vi "Alarma_Auto.vi"() -> ()   [LabVIEW 2020]
panel:
  in  "Boton3":bool
  out "Alarma":bool
  in  "Boton2":bool
  in  "Boton1":bool
  # "Compuertas Logicas"
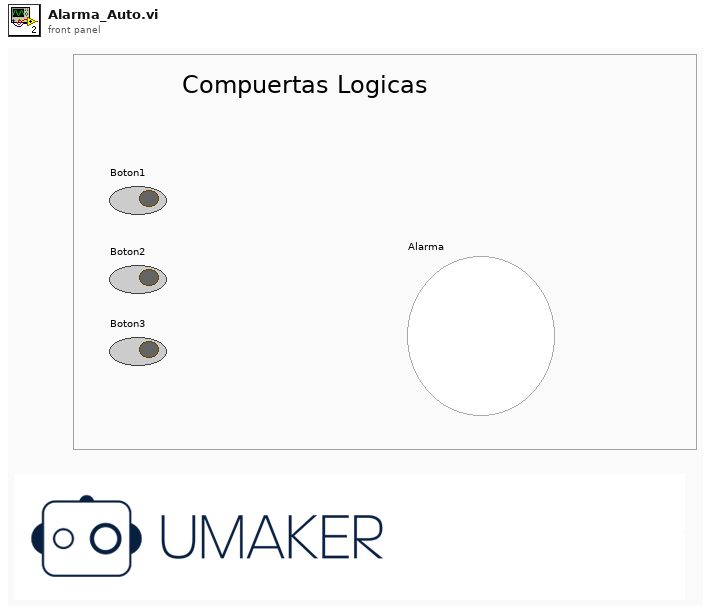
[diagram p1: front panel]
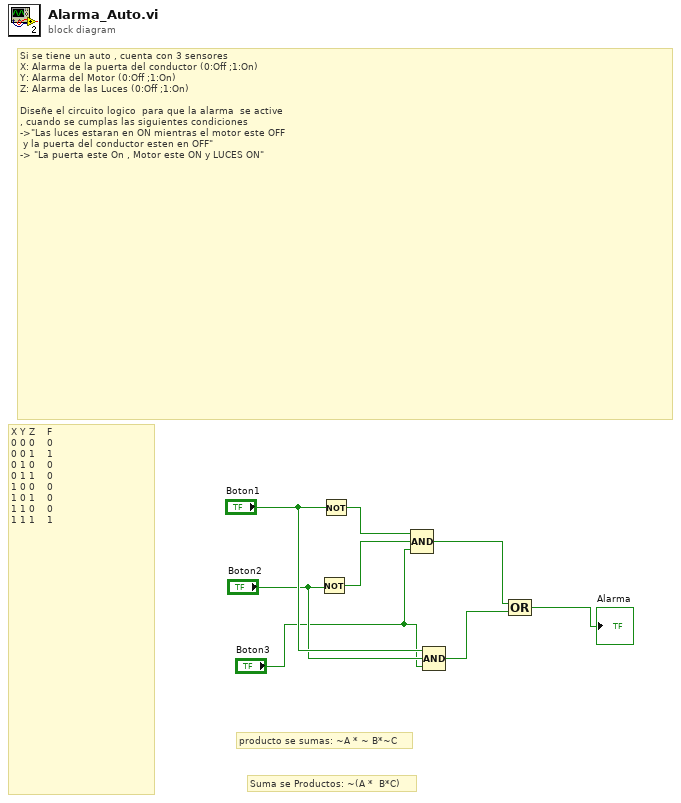
[diagram p0: block diagram]
diagram:
  # "Suma se Productos: ~(A *  B*C)"
  # "producto se sumas: ~A * ~ B*~C"
  # "X Y Z    F\n0 0 0    0   \n0 0 1    1\n0 1 0    0\n0 1 1    0\n1 0 0    0\n1 0 1    0\n1 1 0    0\n1 1 1    1"
  # "Si se tiene un auto , cuenta con 3 sensores\nX: Alarma de la puerta del conductor (0:Off ;1:On)\nY: Alarma del Motor (0:Off ;1:On)\nZ: Alarma de las Luces (0:Off ;1:On)\n\nDiseñe el circuito logico  para que la alarma  se active  \n, cuando se cumplas las siguientes condiciones\n->\"Las luces estaran en ON mientras el motor este OFF\n y la puerta del conductor esten en OFF\"\n-> \"La puerta este On , Motor este ON y LUCES ON\""
  n1 = Not(x="Boton2") -> (.not. x?=w7:bool)
  n2 = Not(x="Boton1") -> (.not. x?=w8:bool)
  n3 = Compound Arithmetic op=AND(w8, w7, "Boton3") -> (w2:bool)
  n4 = Compound Arithmetic op=AND("Boton1", "Boton2", "Boton3") -> (w3:bool)
  n5 = Compound Arithmetic op=OR(w2, w3) -> (→"Alarma":bool)
